vi "Read.vi"(7 "Byte Array as Blobs":bool=TRUE, 8 "Error In":errorcluster, 10 "Types and Defaults":variant, 11 "Reader In":refnum<class "Reader.lvclass">) -> (0 "Error Out":errorcluster, 2 "Value":variant, 3 "Reader Out":refnum<class "Reader.lvclass">)   [LabVIEW 2018, in "Toolkit.lvlib"]
doc: "Recursively reads MessagePack data and decodes based on the supplied type."
uses:
  Toolkit.lvlib
  Public/Reader/Reader.lvclass
  Public/Reader/Reader.lvclass/Reader.ctl
  <vilib>/Utility/Data Type/Type Definitions/Data Type.ctl
  Public/Reader/Private/Handle Error.vi
  Public/Reader/Public/Raw/Read Bytes.vi
  Public/Reader/Private/Read Bytes by Value.vi
  Public/Reader/Public/Status/Read Status.vi
  Public/Reader/Public/Status/Read Status Message.vi
  Public/Reader/Public/Status/Read Is Error.vi
  Public/Reader/Private/Read Nil by Value.vi
  Public/Utility/Status Code.vi
  <vilib>/Utility/error.llb/Error Cluster From Error Code.vi
  Public/Reader/Public/String/Begin Str.vi
  Public/Reader/Private/Begin Str by Value.vi
  Public/Reader/Public/String/End Str.vi
  Public/Reader/Private/End Str by Value.vi
  Public/Reader/Private/Begin Array by Value.vi
  Public/Reader/Private/End Array by Value.vi
  Public/Reader/Public/Binary/Begin Bin.vi
  Public/Reader/Private/Begin Bin by Value.vi
  Public/Reader/Public/Binary/End Bin.vi
  Public/Reader/Private/End Bin by Value.vi
  Public/Reader/Private/Begin Map by Value.vi
  Public/Reader/Private/End Map by Value.vi
  <vilib>/Utility/Data Type/NI_Data Type.lvlib
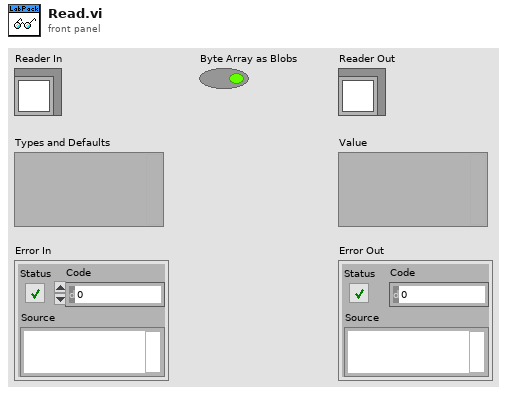
[diagram p1: front panel]
types:
  T1 = typedef "NI_Data Type.lvlib/Data Type.ctl" = enum8{"Invalid Type", "Void", "I8", "I16", "I32", "I64", "U8", "U16", "U32", "U64", "Single Float", "Double Float", "Extended Float", "Single Complex", "Double Complex", "Extended Complex", "Enum U8", "Enum U16", "Enum U32", "Enum U64", "Single Float With Unit", "Double Float With Unit", "Extended Float With Unit", "Single Complex with Unit", "Double Complex with Unit", "Extended Complex with Unit", "Boolean", "String", "Path", "Picture", "Tag", "Array", "Cluster", "Variant", "LV Variant", "Waveform", "Timestamp", "Digital Waveform", "Digital Data", "ExpressData", "Refnum", "External Data", "VI", "Poly VI", "LabVIEW Class Instance", "Fixed Point"}
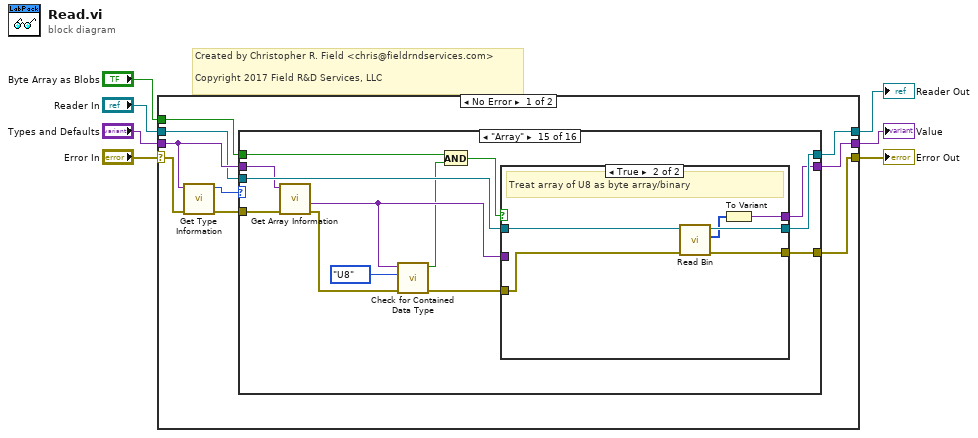
[diagram p0: block diagram]
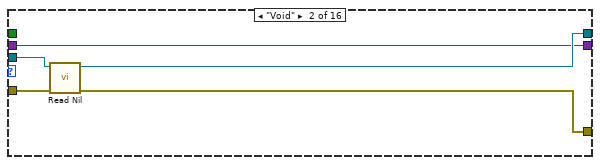
[diagram p3: hidden frame]
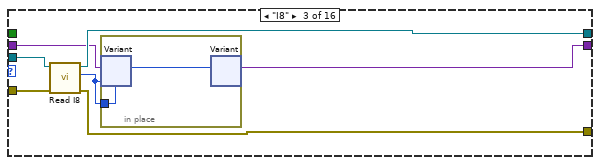
[diagram p4: hidden frame]
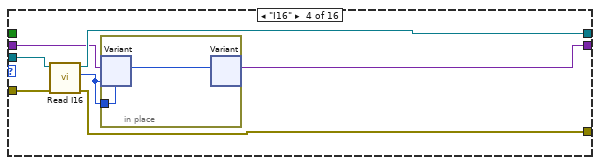
[diagram p5: hidden frame]
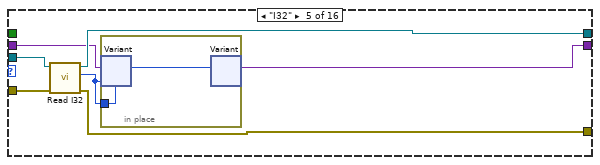
[diagram p6: hidden frame]
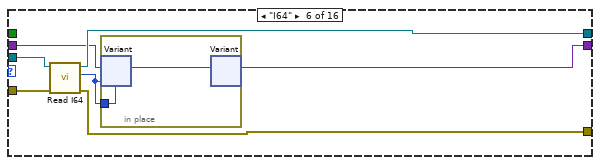
[diagram p7: hidden frame]
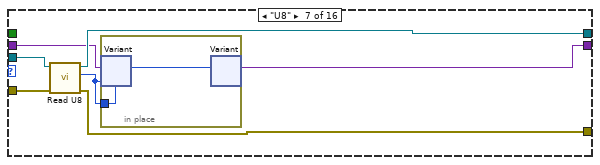
[diagram p8: hidden frame]
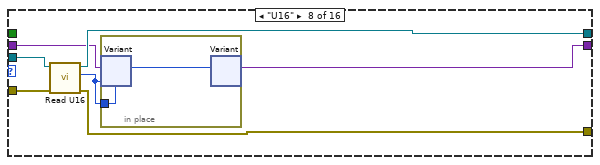
[diagram p9: hidden frame]
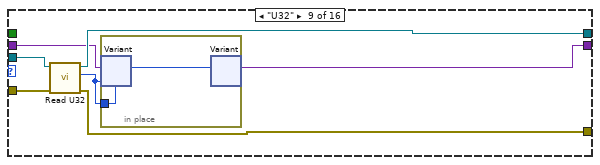
[diagram p10: hidden frame]
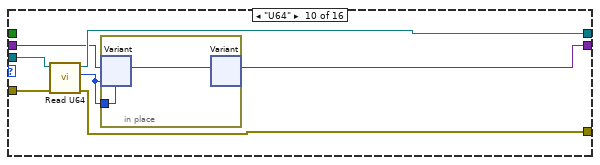
[diagram p11: hidden frame]
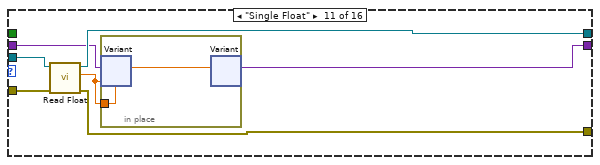
[diagram p12: hidden frame]
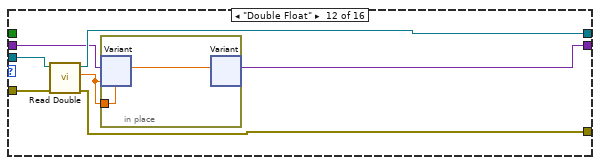
[diagram p13: hidden frame]
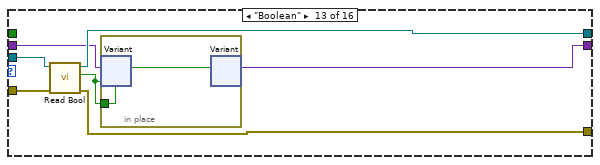
[diagram p14: hidden frame]
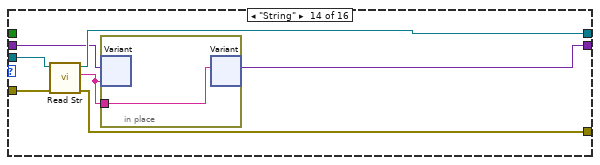
[diagram p15: hidden frame]
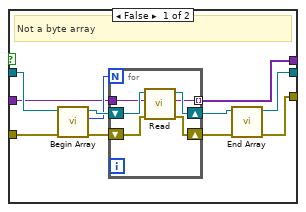
[diagram p16: hidden frame]
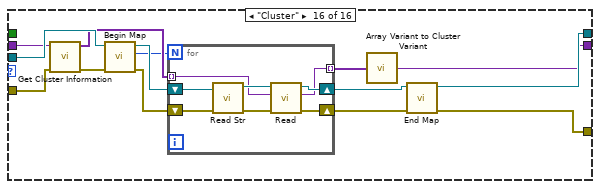
[diagram p17: hidden frame]
diagram:
  # "Created by Christopher R. Field <chris@fieldrndservices.com>\n\nCopyright 2017 Field R&D Services, LLC"
  n1 = case shown="No Error" "Error In" {
    selector: "Error In" -> [w13 w181]
    tunnel: "Types and Defaults" -> [w16 w179]
    tunnel: [w9 w181] -> w6
    tunnel: "Reader In" -> [w12 w180]
    tunnel: [w10 w180] -> w3
    tunnel: [w11 w179] -> w2
    tunnel: "Byte Array as Blobs" -> [w8 _]
    frame No Error {
      n2 = call <vilib>:"Get Type Information.vi"("error in (no error)"=w13, "Variant"=w16) -> ("error out"=w15:errorcluster, "Type"=w14:T1)  [unwired: 5 in, 3 out]
      n3 = case shown="\"Array\"" w14 {
        tunnel: w15 -> [w19 w24 w31 w39 w47 w55 w63 w71 w79 w87 w95 w103 w111 w119 w130 w164]
        tunnel: [w19 w23 w30 w38 w46 w54 w62 w70 w78 w86 w94 w102 w110 w118 w131 w170] -> w9
        tunnel: w16 -> [w17 w20 w27 w35 w42 w51 w59 w67 w75 w82 w90 w99 w106 w115 w129 w162]
        tunnel: w12 -> [w18 w22 w29 w37 w45 w53 w61 w69 w77 w85 w93 w101 w109 w117 w133 w165]
        tunnel: [w18 w21 w28 w36 w44 w52 w60 w68 w76 w84 w92 w100 w108 w116 w132 w166] -> w10
        tunnel: [w17 w20 w25 w34 w41 w50 w58 w66 w74 w81 w89 w98 w105 w114 w121 w157] -> w11
        tunnel: w8 -> [_ _ _ _ _ _ _ _ _ _ _ _ _ _ w122 _]
        frame "Invalid Type", Default {
        }
        frame "Void" {
          n4 = call-poly "Read Nil.vi"("Error In"=w24, "Reader In"=w22) -> ("Error Out"=w23:errorcluster, "Reader Out"=w21:refnum<class "Reader.lvclass">)  [unwired: 8 in]
        }
        frame "I8" {
          n5 = call "Read I8.vi"("Error In"=w31, "Reader In"=w29) -> ("Error Out"=w30:errorcluster, "Value"=w26:i8, "Reader Out"=w28:refnum<class "Reader.lvclass">)  [unwired: 7 in]
          n6 = in-place {
            in-place-border: w26 -> [w32]
            n7 = in-place-variant #1(w27, w26) -> ()  [unwired: 2 out]
            n8 = in-place-variant #1(w32) -> (w25:variant)  [unwired: 1 out]
          }
        }
        frame "I16" {
          n9 = call "Read I16.vi"("Error In"=w39, "Reader In"=w37) -> ("Error Out"=w38:errorcluster, "Value"=w33:i16, "Reader Out"=w36:refnum<class "Reader.lvclass">)  [unwired: 7 in]
          n10 = in-place {
            in-place-border: w33 -> [w40]
            n11 = in-place-variant #2(w35, w33) -> ()  [unwired: 2 out]
            n12 = in-place-variant #2(w40) -> (w34:variant)  [unwired: 1 out]
          }
        }
        frame "I32" {
          n13 = call "Read I32.vi"("Error In"=w47, "Reader In"=w45) -> ("Error Out"=w46:errorcluster, "Value"=w43:i32, "Reader Out"=w44:refnum<class "Reader.lvclass">)  [unwired: 7 in]
          n14 = in-place {
            in-place-border: w43 -> [w48]
            n15 = in-place-variant #3(w42, w43) -> ()  [unwired: 2 out]
            n16 = in-place-variant #3(w48) -> (w41:variant)  [unwired: 1 out]
          }
        }
        frame "I64" {
          n17 = call "Read I64.vi"("Error In"=w55, "Reader In"=w53) -> ("Error Out"=w54:errorcluster, "Value"=w49:i64, "Reader Out"=w52:refnum<class "Reader.lvclass">)  [unwired: 7 in]
          n18 = in-place {
            in-place-border: w49 -> [w56]
            n19 = in-place-variant #4(w51, w49) -> ()  [unwired: 2 out]
            n20 = in-place-variant #4(w56) -> (w50:variant)  [unwired: 1 out]
          }
        }
        frame "U8" {
          n21 = call "Read U8.vi"("Error In"=w63, "Reader In"=w61) -> ("Error Out"=w62:errorcluster, "Value"=w57:u8, "Reader Out"=w60:refnum<class "Reader.lvclass">)  [unwired: 7 in]
          n22 = in-place {
            in-place-border: w57 -> [w64]
            n23 = in-place-variant #5(w59, w57) -> ()  [unwired: 2 out]
            n24 = in-place-variant #5(w64) -> (w58:variant)  [unwired: 1 out]
          }
        }
        frame "U16" {
          n25 = call "Read U16.vi"("Error In"=w71, "Reader In"=w69) -> ("Error Out"=w70:errorcluster, "Value"=w65:u16, "Reader Out"=w68:refnum<class "Reader.lvclass">)  [unwired: 7 in]
          n26 = in-place {
            in-place-border: w65 -> [w72]
            n27 = in-place-variant #6(w67, w65) -> ()  [unwired: 2 out]
            n28 = in-place-variant #6(w72) -> (w66:variant)  [unwired: 1 out]
          }
        }
        frame "U32" {
          n29 = call "Read U32.vi"("Error In"=w79, "Reader In"=w77) -> ("Error Out"=w78:errorcluster, "Value"=w73:u32, "Reader Out"=w76:refnum<class "Reader.lvclass">)  [unwired: 7 in]
          n30 = in-place {
            in-place-border: w73 -> [w80]
            n31 = in-place-variant #7(w75, w73) -> ()  [unwired: 2 out]
            n32 = in-place-variant #7(w80) -> (w74:variant)  [unwired: 1 out]
          }
        }
        frame "U64" {
          n33 = call "Read U64.vi"("Error In"=w87, "Reader In"=w85) -> ("Error Out"=w86:errorcluster, "Value"=w83:u64, "Reader Out"=w84:refnum<class "Reader.lvclass">)  [unwired: 7 in]
          n34 = in-place {
            in-place-border: w83 -> [w88]
            n35 = in-place-variant #8(w82, w83) -> ()  [unwired: 2 out]
            n36 = in-place-variant #8(w88) -> (w81:variant)  [unwired: 1 out]
          }
        }
        frame "Single Float" {
          n37 = call "Read Float.vi"("Error In"=w95, "Reader In"=w93) -> ("Error Out"=w94:errorcluster, "Value"=w91:sgl, "Reader Out"=w92:refnum<class "Reader.lvclass">)  [unwired: 7 in]
          n38 = in-place {
            in-place-border: w91 -> [w96]
            n39 = in-place-variant #9(w90, w91) -> ()  [unwired: 2 out]
            n40 = in-place-variant #9(w96) -> (w89:variant)  [unwired: 1 out]
          }
        }
        frame "Double Float" {
          n41 = call "Read Double.vi"("Error In"=w103, "Reader In"=w101) -> ("Error Out"=w102:errorcluster, "Value"=w97:dbl, "Reader Out"=w100:refnum<class "Reader.lvclass">)  [unwired: 7 in]
          n42 = in-place {
            in-place-border: w97 -> [w104]
            n43 = in-place-variant #10(w99, w97) -> ()  [unwired: 2 out]
            n44 = in-place-variant #10(w104) -> (w98:variant)  [unwired: 1 out]
          }
        }
        frame "Boolean" {
          n45 = call "Read Bool.vi"("Error In"=w111, "Reader In"=w109) -> ("Error Out"=w110:errorcluster, "Value"=w107:bool, "Reader Out"=w108:refnum<class "Reader.lvclass">)  [unwired: 7 in]
          n46 = in-place {
            in-place-border: w107 -> [w112]
            n47 = in-place-variant #11(w106, w107) -> ()  [unwired: 2 out]
            n48 = in-place-variant #11(w112) -> (w105:variant)  [unwired: 1 out]
          }
        }
        frame "String" {
          n49 = call "Read Str.vi"("Error In"=w119, "Reader In"=w117) -> ("Error Out"=w118:errorcluster, "Value"=w113:string, "Reader Out"=w116:refnum<class "Reader.lvclass">)  [unwired: 7 in]
          n50 = in-place {
            in-place-border: w113 -> [w120]
            n51 = in-place-variant #12(w115, w113) -> ()  [unwired: 2 out]
            n52 = in-place-variant #12(w120) -> (w114:variant)  [unwired: 1 out]
          }
        }
        frame "Array" {
          n53 = call <vilib>:"Get Array Information.vi"("error in (no error)"=w130, "Variant"=w129) -> ("error out"=w127:errorcluster, "Array Element Data Type"=w128:variant)  [unwired: 6 in, 2 out]
          n54 = call <vilib>:"Check for Contained Data Type.vi"("error in (no error)"=w127, "Data Type to Find"=Data_Type."U8", "Variant"=w128) -> ("error out"=w126:errorcluster, "Contains Data Type to Find?"=w124:bool)  [unwired: 7 in]
          n55 = And(x=w122, y=w124) -> (x .and. y?=w123:bool)
          n56 = case shown="True" w123 {
            tunnel: w133 -> [w144 w156]
            tunnel: [w143 w155] -> w132
            tunnel: [w142 w151] -> w131
            tunnel: w128 -> [w136 _]
            tunnel: w126 -> [w135 w152]
            tunnel: [w134 w153] -> w121
            frame False {
              # "Not a byte array"
              n57 = call-poly "Begin Array.vi"("Error In"=w135, "Reader In"=w144) -> ("Error Out"=w138:errorcluster, "Count"=w137:u32, "Reader Out"=w139:refnum<class "Reader.lvclass">)  [unwired: 7 in]
              n58 = for {
                N: w137 -> [_]
                shift-right: [w147] -> w141
                shift-left: w139 -> [w148]
                shift-right: [w150] -> w140
                shift-left: w138 -> [w149]
                tunnel: [w146] -> w134 mode=indexing
                tunnel: w136 -> [w145]
                n59 = call "Read.vi"("Error In"=w149, "Types and Defaults"=w145, "Reader In"=w148) -> ("Error Out"=w150:errorcluster, "Value"=w146:variant, "Reader Out"=w147:refnum<class "Reader.lvclass">)  [unwired: 6 in]
              }
              n60 = call-poly "End Array.vi"("Error In"=w140, "Reader In"=w141) -> ("Error Out"=w142:errorcluster, "Reader Out"=w143:refnum<class "Reader.lvclass">)  [unwired: 8 in]
            }
            frame True {
              # "Treat array of U8 as byte array/binary"
              n61 = call "Read Bin.vi"("Error In"=w152, "Reader In"=w156) -> ("Error Out"=w151:errorcluster, "Value"=w154:u8[], "Reader Out"=w155:refnum<class "Reader.lvclass">)  [unwired: 7 in]
              n62 = To Variant(anything=w154) -> (Variant=w153:variant)
            }
          }
        }
        frame "Cluster" {
          n63 = call <vilib>:"Get Cluster Information.vi"("error in (no error)"=w164, "Variant"=w162) -> ("error out"=w161:errorcluster, "Cluster Elements"=w163:variant[])  [unwired: 8 in]
          n64 = call-poly "Begin Map.vi"("Error In"=w161, "Reader In"=w165) -> ("Error Out"=w168:errorcluster, "Count"=w159:u32, "Reader Out"=w169:refnum<class "Reader.lvclass">)  [unwired: 7 in]
          n65 = for {
            N: w159 -> [_]
            shift-right: [w175] -> w167
            shift-left: w169 -> [w177]
            shift-right: [w173] -> w160
            shift-left: w168 -> [w178]
            tunnel: [w174] -> w158 mode=indexing
            tunnel: w163 -> [w172] mode=indexing
            n66 = call "Read Str.vi"("Error In"=w178, "Reader In"=w177) -> ("Error Out"=w171:errorcluster, "Reader Out"=w176:refnum<class "Reader.lvclass">)  [unwired: 7 in, 1 out]
            n67 = call "Read.vi"("Error In"=w171, "Types and Defaults"=w172, "Reader In"=w176) -> ("Error Out"=w173:errorcluster, "Value"=w174:variant, "Reader Out"=w175:refnum<class "Reader.lvclass">)  [unwired: 6 in]
          }
          n68 = call "Array Variant to Cluster Variant.vi"("Array"=w158) -> ("Cluster"=w157:variant)
          n69 = call-poly "End Map.vi"("Error In"=w160, "Reader In"=w167) -> ("Error Out"=w170:errorcluster, "Reader Out"=w166:refnum<class "Reader.lvclass">)  [unwired: 8 in]
        }
      }
    }
    frame Error {
    }
  }
  "Error Out" <- w6
  "Reader Out" <- w3
  "Value" <- w2
